vi "ma_sml_Cascaded Decimation Filter.vi"   [LabVIEW 2020, in "NI_MAPro.lvlib"]
uses:
  NI_MAPro.lvlib
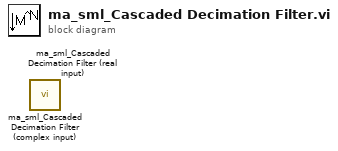
[diagram p0: block diagram]
diagram:
  n1 = call "ma_sml_Cascaded Decimation Filter (complex input).vi"() -> ()  [unwired: 3 in, 1 out]
  n2 = call "ma_sml_Cascaded Decimation Filter (real input).vi"() -> ()  [unwired: 3 in, 1 out]
